vi "Check sweep timing.vi"(8 "error in (no error)":errorcluster, 10 "Tolerance (s)":dbl, 11 "DAQOrcaFlash in":refnum<class "DAQOrcaFlash.lvclass">) -> (0 "error out":errorcluster, 2 "out of time?":bool, 3 "DAQOrcaFlash out":refnum<class "DAQOrcaFlash.lvclass">)   [LabVIEW 2012, in "DAQOrcaFlash.lvclass"]
uses:
  DAQOrcaFlash.lvclass
  DAQOrcaFlash.lvclass/DAQOrcaFlash.ctl
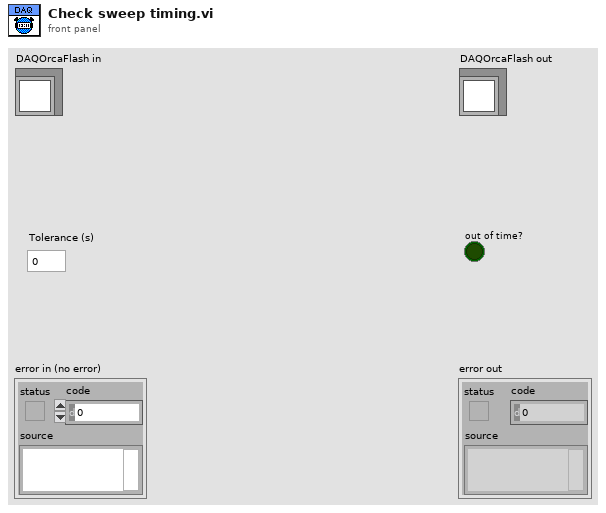
[diagram p1: front panel]
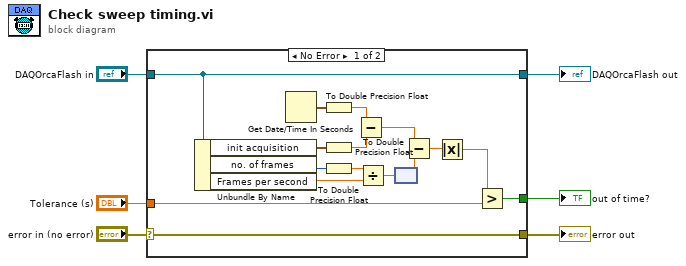
[diagram p0: block diagram]
diagram:
  n1 = case shown="No Error" "error in (no error)" {
    selector: "error in (no error)" -> [w22 w24]
    tunnel: [w22 w24] -> w5
    tunnel: [w21 w23] -> w3
    tunnel: "DAQOrcaFlash in" -> [w21 w23]
    tunnel: "Tolerance (s)" -> [w8 _]
    tunnel: [w7 _] -> w1
    frame No Error {
      n2 = Unbundle By Name(w21) -> ("init acquisition"=w17:timestamp, "no. of frames"=w20:i32, "Frames per second"=w19:dbl[unit])
      n3 = Get Date/Time In Seconds() -> (seconds since 1Jan1904=w16:timestamp)
      n4 = To Double Precision Float(number=w16) -> (double precision float=w15:dbl)
      n5 = To Double Precision Float(number=w17) -> (double precision float=w14:dbl)
      n6 = To Double Precision Float(number=w20) -> (double precision float=w18:dbl)
      n7 = Subtract(x=w15, y=w14) -> (x-y=w13:dbl)
      n8 = Divide(x=w18, y=w19) -> (x/y=w12:dbl[unit])
      n9 = node(w12) -> (w11:dbl)
      n10 = Subtract(x=w13, y=w11) -> (x-y=w10:dbl)
      n11 = Absolute Value(x=w10) -> (abs(x)=w9:dbl)
      n12 = Greater?(x=w9, y=w8) -> (0:w7:bool)
    }
    frame Error {
    }
  }
  "error out" <- w5
  "DAQOrcaFlash out" <- w3
  "out of time?" <- w1
